vi "ToolBarButtonDraw_undo.vi"(6 "Color":u32(colorbox), 7 "undo size":i32=5, 10 "rect":T1, 11 "Pict IN":picture) -> (3 "Pict OUT":picture)   [LabVIEW 2020, in "Sgraph_lib_V1.lvlib" / "Gviewer.lvclass"]
doc: "Draw Undo icon with memory depth in button bar"
uses:
  Gviewer.lvclass
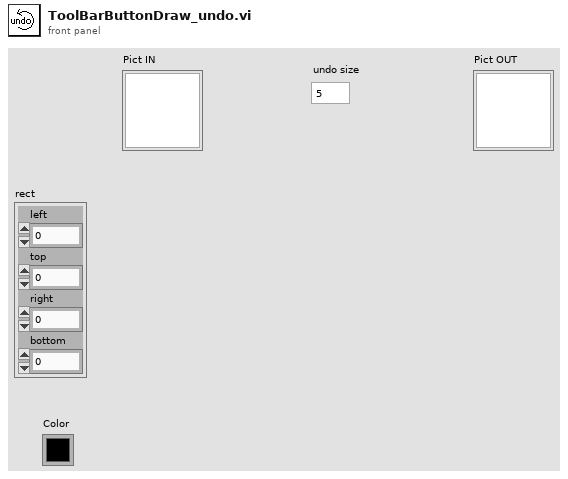
[diagram p1: front panel]
types:
  T1 = cluster{"left":i16, "top":i16, "right":i16, "bottom":i16}
  T2 = cluster{"Font Name:":string, "Size":i16, "Strikeout?":bool, "Italic?":bool, "Underline?":bool, "Outline?":bool, "Shadow?":bool, "Bold?":bool}
  T3 = enum16{"User-specified Font", "Application Font", "System Font", "Dialog Font"}
  T4 = cluster{"horizontal":enum16{"left", "center", "right"}, "vertical":enum16{"top", "center", "bottom"}}
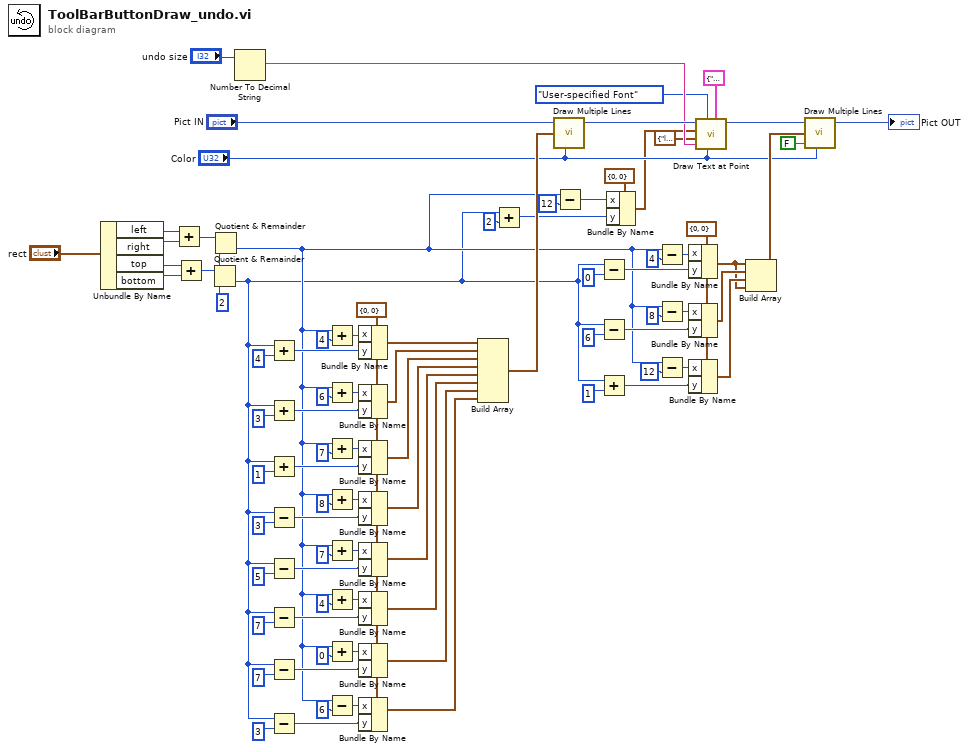
[diagram p0: block diagram]
diagram:
  w20 = cluster{"x":i16, "y":i16} {"x"=0, "y"=0}
  w37 = cluster{"x":i16, "y":i16} {"x"=0, "y"=0}
  w80 = i16 2 ("y")
  n1 = Unbundle By Name("rect") -> ("left"=w86:i16, "right"=w85:i16, "top"=w84:i16, "bottom"=w83:i16)
  n2 = Add(x=w86, y=w85) -> (x+y=w82:i16)
  n3 = Add(x=w84, y=w83) -> (x+y=w81:i16)
  n4 = Quotient & Remainder(x=w81, y=w80) -> (floor(x/y)=w2:i16)  [unwired: 1 out]
  n5 = Quotient & Remainder(x=w82, y=w80) -> (floor(x/y)=w6:i16)  [unwired: 1 out]
  n6 = Number To Decimal String(number="undo size") -> (decimal integer string=w12:string)  [unwired: 1 in]
  n7 = Add(x=w2, y=i16 4) -> (x+y=w72:i16)
  n8 = Add(x=w2, y=i16 3) -> (x+y=w69:i16)
  n9 = Add(x=w2, y=i16 1) -> (x+y=w65:i16)
  n10 = Subtract(x=w2, y=i16 3) -> (x-y=w59:i16)
  n11 = Subtract(x=w2, y=i16 5) -> (x-y=w55:i16)
  n12 = Subtract(x=w2, y=i16 7) -> (x-y=w42:i16)
  n13 = Subtract(x=w2, y=i16 7) -> (x-y=w46:i16)
  n14 = Subtract(x=w2, y=i16 3) -> (x-y=w39:i16)
  n15 = Add(x=w6, y=i16 4) -> (x+y=w78:i16)
  n16 = Add(x=w6, y=i16 6) -> (x+y=w68:i16)
  n17 = Add(x=w6, y=i16 7) -> (x+y=w66:i16)
  n18 = Add(x=w6, y=i16 8) -> (x+y=w58:i16)
  n19 = Add(x=w6, y=i16 7) -> (x+y=w56:i16)
  n20 = Add(x=w6, y=i16 4) -> (x+y=w49:i16)
  n21 = Add(x=w6, y=i16 0) -> (x+y=w47:i16)
  n22 = Subtract(x=w6, y=i16 6) -> (x-y=w38:i16)
  n23 = Bundle By Name(cluster=w37, "x"=w78, "y"=w72) -> (w77:cluster{"x":i16, "y":i16})
  n24 = Bundle By Name(cluster=w37, "x"=w68, "y"=w69) -> (w67:cluster{"x":i16, "y":i16})
  n25 = Bundle By Name(cluster=w37, "x"=w66, "y"=w65) -> (w62:cluster{"x":i16, "y":i16})
  n26 = Bundle By Name(cluster=w37, "x"=w58, "y"=w59) -> (w57:cluster{"x":i16, "y":i16})
  n27 = Bundle By Name(cluster=w37, "x"=w56, "y"=w55) -> (w52:cluster{"x":i16, "y":i16})
  n28 = Bundle By Name(cluster=w37, "x"=w49, "y"=w42) -> (w48:cluster{"x":i16, "y":i16})
  n29 = Bundle By Name(cluster=w37, "x"=w47, "y"=w46) -> (w43:cluster{"x":i16, "y":i16})
  n30 = Bundle By Name(cluster=w37, "x"=w38, "y"=w39) -> (w36:cluster{"x":i16, "y":i16})
  n31 = Build Array(w77, w67, w62, w57, w52, w48, w43, w36) -> (w76:cluster{"x":i16, "y":i16}[])
  n32 = Add(x=w2, y=i16 2) -> (x+y=w1:i16)
  n33 = call <vilib>:"Draw Multiple Lines.vi"("picture"="Pict IN", "line endpoints"=w76, "color(black)"="Color") -> ("new picture"=w16:picture)  [unwired: 6 in]
  n34 = Subtract(x=w6, y=i16 12) -> (x-y=w7:i16)
  n35 = Subtract(x=w2, y=i16 0) -> (x-y=w25:i16)
  n36 = Subtract(x=w2, y=i16 6) -> (x-y=w28:i16)
  n37 = Add(x=w2, y=i16 1) -> (x+y=w31:i16)
  n38 = Bundle By Name(cluster=cluster{"x":i16, "y":i16} {"x"=0, "y"=0}, "x"=w7, "y"=w1) -> (w9:cluster{"x":i16, "y":i16})
  n39 = Subtract(x=w6, y=i16 4) -> (x-y=w23:i16)
  n40 = Subtract(x=w6, y=i16 8) -> (x-y=w29:i16)
  n41 = Subtract(x=w6, y=i16 12) -> (x-y=w30:i16)
  n42 = Bundle By Name(cluster=w20, "x"=w23, "y"=w25) -> (w18:cluster{"x":i16, "y":i16})
  n43 = Bundle By Name(cluster=w20, "x"=w29, "y"=w28) -> (w21:cluster{"x":i16, "y":i16})
  n44 = Bundle By Name(cluster=w20, "x"=w30, "y"=w31) -> (w19:cluster{"x":i16, "y":i16})
  n45 = call <vilib>:"Draw Text at Point.vi"("[user-specified font]"=T2 {"Font Name:"="Arial", "Size"=11, "Strikeout?"=FALSE, "Italic?"=FALSE, "Underline?"=FALSE, "Outline?"=FALSE, "Shadow?"=FALSE, "Bold?"=FALSE}, "text color(black)"="Color", "desired font(Application)"=T3."User-specified Font", "text"=w12, "alignment(left, top)"=T4 {"horizontal"=enum."left", "vertical"=enum."top"}, "origin"=w9, "picture"=w16) -> ("new picture"=w15:picture)  [unwired: 3 in, 1 out]
  n46 = Build Array(w18, w21, w19, w18) -> (w33:cluster{"x":i16, "y":i16}[])
  n47 = call <vilib>:"Draw Multiple Lines.vi"("picture"=w15, "line endpoints"=w33, "fill?(F)"=FALSE, "color(black)"="Color") -> ("new picture"=→"Pict OUT":picture)  [unwired: 5 in]
